vi "Force update objective calibration settings .vi"(8 "error in (no error)":errorcluster, 10 "Current Calibration Parameters":T1, 11 "Current Objective":string) -> (0 "error out":errorcluster)   [LabVIEW 2020]
uses:
  Calibration/ToolBox/TypeDefs/Current Calibration Parameters.ctl
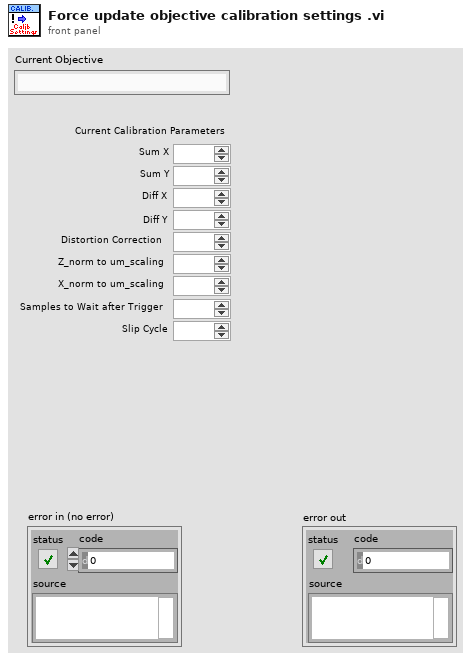
[diagram p1: front panel]
types:
  T1 = typedef "Current Calibration Parameters.ctl" = cluster{"Sum X":dbl, "Sum Y":dbl, "Diff X":dbl, "Diff Y":dbl, "Distortion Correction":dbl, "Z_norm to um_scaling":dbl, "X_norm to um_scaling":dbl, "Samples to Wait after Trigger":dbl, "Slip Cycle":dbl}
  T2 = enum16{"Initialise", "Load from file", "Save to file", "Read", "Write"}
  T3 = typedef "Calibration config.ctl" = cluster{"Current Objective":string, "Objective Settings":T4[], "PreChirper Values Preset ?":bool, "PreChirper Settings":T5[], "PreChirper Constants":T6}
  T4 = typedef "Objective Config.ctl" = cluster{"Name":string, "Sum X":dbl, "Sum Y":dbl, "Diff X":dbl, "Diff Y":dbl, "Distortion Correction":dbl, "Z_norm to um_scaling":dbl, "X_norm to um_scaling":dbl, "Calibrated Wavelength":dbl}
  T5 = typedef "Prechirper Cal Config.ctl" = cluster{"Wavelength":i32, "Prism 1":i32, "Prism 2":i32}
  T6 = typedef "PreChirper constants.ctl" = cluster{"a 1":i32, "b 1":i32, "c 1":i32, "a 2":i32, "b 2":i32, "c 2":i32, "lmin":i32, "lmax":i32}
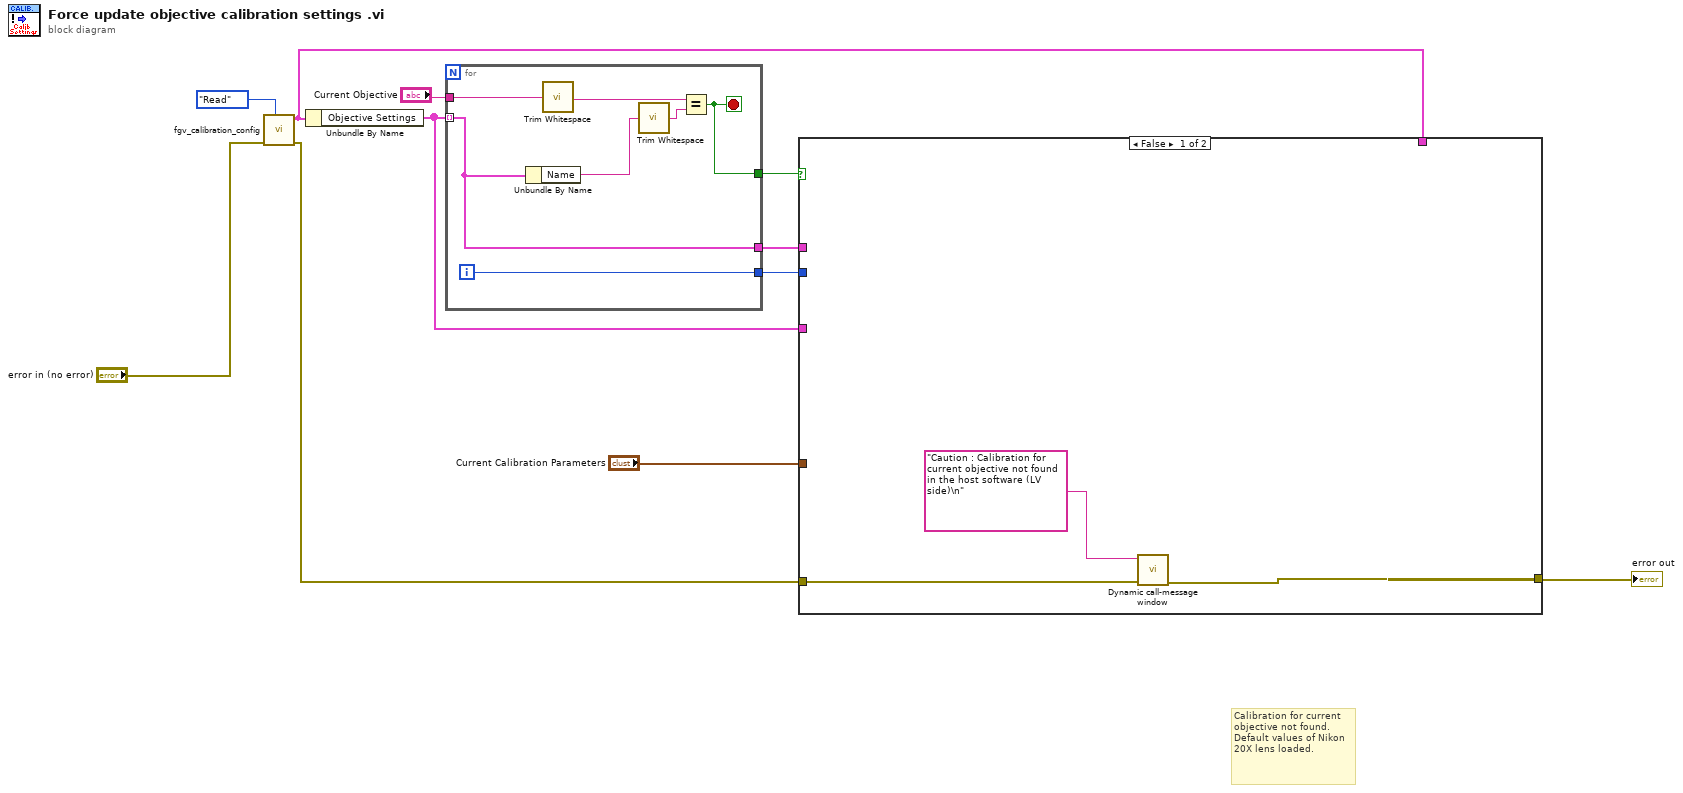
[diagram p0: block diagram]
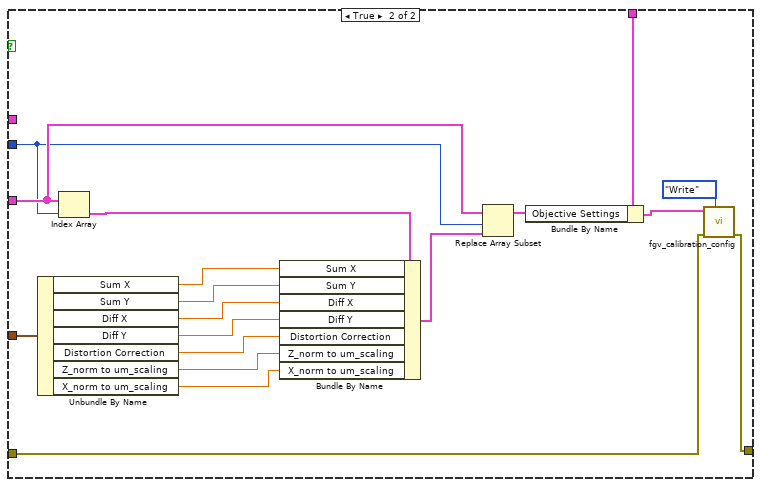
[diagram p2: hidden frame]
diagram:
  # "Calibration for current objective not found.\nDefault values of Nikon 20X lens loaded."
  n1 = call "fgv_calibration_config.vi"("Cal config ops"=T2."Read", "error in (no error)"="error in (no error)") -> ("error out"=w8:errorcluster, "Config cluster OUT"=w1:T3)  [unwired: 7 in, 1 out]
  n2 = Unbundle By Name(w1) -> ("Objective Settings"=w3:T4[])
  n3 = for {
    tunnel: "Current Objective" -> [w18]
    tunnel: w3 -> [w13] mode=indexing
    tunnel: [w14] -> w10
    tunnel: [w13] -> w5
    tunnel: [w12] -> w4
    i -> [w12]
    stop <- w14 stop-if-true
    n4 = Unbundle By Name(w13) -> ("Name"=w17:string)
    n5 = call <vilib>:"Trim Whitespace.vi"("string"=w18) -> ("trimmed string"=w15:string)  [unwired: 1 in]
    n6 = call <vilib>:"Trim Whitespace.vi"("string"=w17) -> ("trimmed string"=w16:string)  [unwired: 1 in]
    n7 = Equal?(x=w15, y=w16) -> (x = y?=w14:bool)
  }
  n8 = case shown="False" w10 {
    tunnel: w8 -> [w21 w23]
    tunnel: [w20 w22] -> w7
    tunnel: w5 -> [_ _]
    tunnel: w4 -> [_ w29]
    tunnel: w3 -> [_ w30]
    tunnel: "Current Calibration Parameters" -> [_ w38]
    tunnel: w1 -> [_ w27]
    frame False {
      n9 = call "Dynamic call-message window.vi"("error in (no error)"=w21, "Message"="Caution : Calibration for current objective not found in the host software (LV side)\n") -> ("error out"=w20:errorcluster)  [unwired: 9 in]
    }
    frame True {
      n10 = Unbundle By Name(w38) -> ("Sum X"=w37:dbl, "Sum Y"=w36:dbl, "Diff X"=w35:dbl, "Diff Y"=w34:dbl, "Distortion Correction"=w33:dbl, "Z_norm to um_scaling"=w32:dbl, "X_norm to um_scaling"=w31:dbl)
      n11 = Index Array(array=w30, index=w29) -> (element=w39:T4)
      n12 = Bundle By Name(cluster=w39, "Sum X"=w37, "Sum Y"=w36, "Diff X"=w35, "Diff Y"=w34, "Distortion Correction"=w33, "Z_norm to um_scaling"=w32, "X_norm to um_scaling"=w31) -> (w28:T4)
      n13 = Replace Array Subset(array=w30, new element=w28, index=w29) -> (w26:T4[])
      n14 = Bundle By Name(cluster=w27, "Objective Settings"=w26) -> (w24:T3)
      n15 = call "fgv_calibration_config.vi"("Cal config ops"=T2."Write", "error in (no error)"=w23, "Config cluster IN"=w24) -> ("error out"=w22:errorcluster)  [unwired: 6 in, 2 out]
    }
  }
  "error out" <- w7
